vi "CopyFromDVR.vi"(8 "error in":errorcluster, 11 "node in":refnum<data-value>) -> (0 "error out":errorcluster, 2 "NISE_CEF_Node out":refnum<class "NISE_CEF_Node.lvclass">, 3 "node out":refnum<data-value>)   [LabVIEW 2013, in "NISE_CEF_Node.lvclass"]
uses:
  NISE_CEF_Node.lvclass
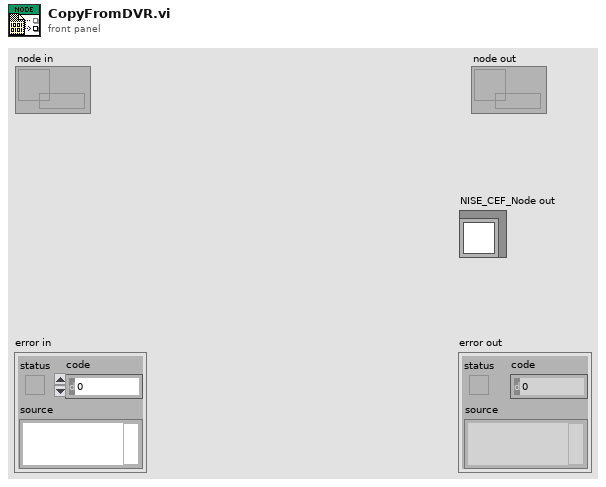
[diagram p1: front panel]
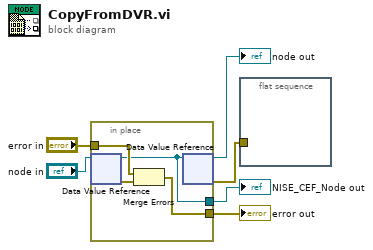
[diagram p0: block diagram]
diagram:
  n1 = in-place {
    in-place-border: "error in" -> [w10]
    in-place-border: [w9] -> w5
    in-place-border: [w7] -> w1
    n2 = in-place-dvr #1("node in") -> (w7:refnum<class "NISE_CEF_Node.lvclass">, w8:errorcluster)
    n3 = Merge Errors(w10, w8) -> (w9:errorcluster)
    n4 = in-place-dvr #1(w7) -> (→"node out":refnum<data-value>, w2:errorcluster)
  }
  "error out" <- w5
  "NISE_CEF_Node out" <- w1
  n5 = flat-sequence {
    tunnel: w2 -> [_]
    frame #0 {
    }
  }
